vi "GetMetadataKey.vi"(7 "DLL path":path, 8 "error in (no error)":errorcluster, 10 "index":i32, 11 "session id in":i32) -> (0 "error out":errorcluster, 1 "MetadataKey":string, 3 "session id out":i32)   [LabVIEW 2017, in "ONNX Class Library.lvlib"]
doc: "/**\n * @brief Получить ключ метаданных по индексу\n * \n * @param sessionId [IN] ID сессии\n * @param index [IN] Индекс метаданных (0-based)\n * @param buffer [OUT] Буфер для строки с ключом\n * @param bufferSize [IN] Размер буфера (рекомендуется 256)\n * \n * @return int32: 0 при успехе\n * @return int32: -1 если индекс неверен\n * \n * @example Ключи: \"producer_name\", \"graph_name\", \"model_version\"\n */\nint GetMetadataKey(int sessionId, int index, char* buffer, int bufferSize);"
uses:
  ONNX Class Library.lvlib
panel:
  out "bufferSize":i32
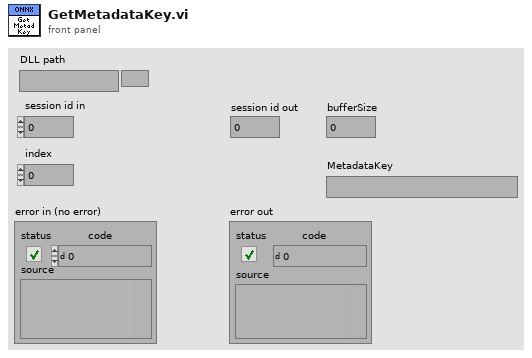
[diagram p1: front panel]
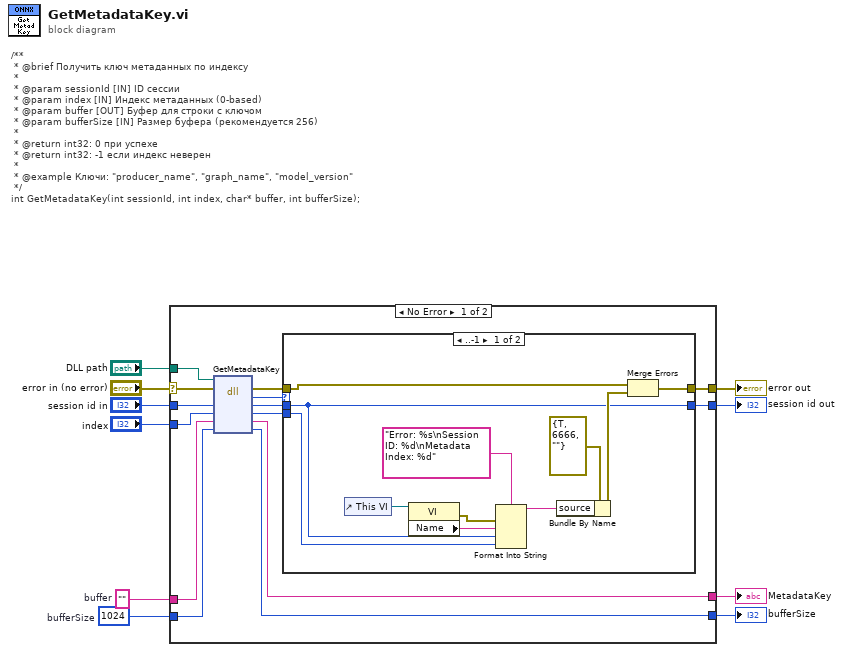
[diagram p0: block diagram]
diagram:
  w7 = 1024  # bufferSize
  w9 = ""  # buffer
  # "/**\n * @brief Получить ключ метаданных по индексу\n * \n * @param sessionId [IN] ID сессии\n * @param index [IN] Индекс метаданных (0-based)\n * @param buffer [OUT] Буфер для строки с ключом\n * @param bufferSize [IN] Размер буфера (рекомендуется 256)\n * \n * @return int32: 0 при успехе\n * @return int32: -1 если индекс неверен\n * \n * @example Ключи: \"producer_name\", \"graph_name\", \"model_version\"\n */\nint GetMetadataKey(int sessionId, int index, char* buffer, int bufferSize);"
  n1 = case shown="No Error" "error in (no error)" {
    selector: "error in (no error)" -> [w12 w39]
    tunnel: "index" -> [w24 _]
    tunnel: w9 -> [w23 _]
    tunnel: [w22 _] -> w8
    tunnel: w7 -> [w21 _]
    tunnel: "session id in" -> [w20 w38]
    tunnel: [w19 _] -> w5
    tunnel: [w17 w39] -> w4
    tunnel: [w16 w38] -> w3
    tunnel: "DLL path" -> [w11 _]
    frame No Error {
      n2 = dll-call lib="home/ivan/LabVIEWData/ONNX/Test/libonnx_wrapper/unix64/libonnx_wrapper.so" fn="GetMetadataKey"(path in=w11, error in=w12, "sessionId"=w20, "inputIndex"=w24, "buffer"=w23, "bufferSize"=w21) -> (error out=w18:errorcluster, "return"=w15:i32, "sessionId"=w14:i32, "inputIndex"=w13:i32, "buffer"=w22:string, "bufferSize"=w19:i32)  [unwired: 1 in, 1 out]
      n3 = case shown="..-1" w15 {
        tunnel: w18 -> [w26 w37]
        tunnel: [w27 w37] -> w17
        tunnel: w14 -> [w28 w36]
        tunnel: [w28 w36] -> w16
        tunnel: w13 -> [w25 _]
        frame ..-1 {
          n4 = control-ref of="This VI"() -> (w32:refnum<vi>)
          n5 = property class="VI"(reference=w32) -> (error out=w29:errorcluster, "Name"=w31:string)  [unwired: 1 in, 1 out]
          n6 = Format Into String(format string="Error: %s\nSession ID: %d\nMetadata Index: %d", error in=w29, w31, w28, w25) -> (resulting string=w33:string)  [unwired: 1 in, 1 out]
          n7 = Bundle By Name(cluster=errorcluster {"status"=TRUE, "code"=6666, "source"=""} ("error out"), "source"=w33) -> (w34:errorcluster)
          n8 = Merge Errors(w26, w34) -> (w27:errorcluster)
        }
        frame 0.. {
        }
      }
    }
    frame Error {
    }
  }
  "error out" <- w4
  "session id out" <- w3
  "MetadataKey" <- w8
  "bufferSize" <- w5
